vi "Dual Sonar and Perpendicular Distance.vi"(0 "Sonar Offset":dbl, 1 "Left Sonar Dev Ref":T1, 2 "Sonar Scale":dbl(knob)=103.01876216940353 scale=0.0..120.0, 3 "Radius of Ball":dbl=12.5, 4 "Right Sonar Dev Ref":T1, 5 "ResetSonar":bool) -> (6 "Left":dbl(graph), 7 "Right":dbl(graph), 8 "Perpendicular Distance to Ball":dbl(graph))   [LabVIEW 2013]
uses:
  <vilib>/Rock Robotics/WPI/AnalogChannel/WPI_AnalogChannelDevRef.ctl
  <vilib>/Rock Robotics/SystemInterfaces/Typedef/FPGA_TypedefAnalogModule.ctl
  <vilib>/Rock Robotics/SystemInterfaces/AI/FPGA_AIChannel.ctl
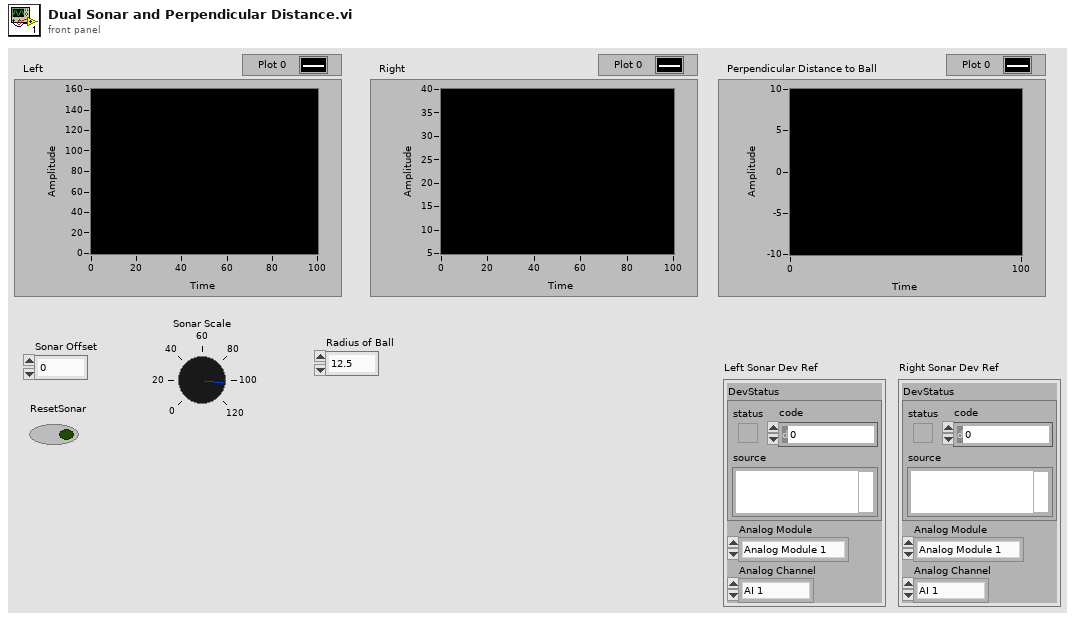
[diagram p1: front panel]
types:
  T1 = typedef "WPI_AnalogChannelDevRef.ctl" = cluster{"DevStatus":errorcluster, "Analog Module":T2, "Analog Channel":T3}
  T2 = typedef "FPGA_TypedefAnalogModule.ctl" = enum16{"Analog Module 1", "Analog Module 2"}
  T3 = typedef "FPGA_AIChannel.ctl" = enum8{"AI 1", "AI 2", "AI 3", "AI 4", "AI 5", "AI 6", "AI 7", "AI 8", "Invalid"}
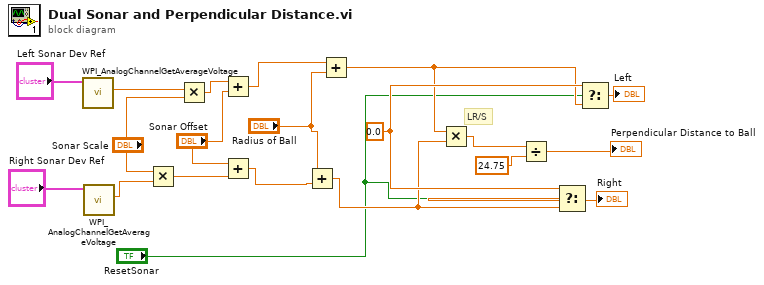
[diagram p0: block diagram]
diagram:
  w18 = 0.0
  # "LR/S"
  n1 = call <vilib>:"WPI_AnalogChannelGetAverageVoltage.vi"("AIDeviceRef"="Left Sonar Dev Ref") -> ("Voltage"=w17:dbl)  [unwired: 8 in, 2 out]
  n2 = call <vilib>:"WPI_AnalogChannelGetAverageVoltage.vi"("AIDeviceRef"="Right Sonar Dev Ref") -> ("Voltage"=w15:dbl)  [unwired: 8 in, 2 out]
  n3 = Multiply(x="Sonar Scale", y=w15) -> (x*y=w12:dbl)
  n4 = Multiply(x=w17, y="Sonar Scale") -> (x*y=w16:dbl)
  n5 = Add(x=w16, y="Sonar Offset") -> (x+y=w11:dbl)
  n6 = Add(x="Sonar Offset", y=w12) -> (x+y=w10:dbl)
  n7 = Add(x="Radius of Ball", y=w10) -> (x+y=w8:dbl)
  n8 = Add(x=w11, y="Radius of Ball") -> (x+y=w9:dbl)
  n9 = Multiply(x=w9, y=w8) -> (x*y=w7:dbl)
  n10 = Divide(x=w7, y=24.75) -> (x/y=→"Perpendicular Distance to Ball":dbl)
  n11 = Select(t=w18, s="ResetSonar", f=w8) -> (s? t:f=→"Right":dbl)
  n12 = Select(t=w18, s="ResetSonar", f=w9) -> (s? t:f=→"Left":dbl)
